vi "VisBx Simulation mit Enum.vi"() -> ()   [LabVIEW 2020, in "Anlagenuebersicht.lvlib"]
uses:
  Anlagenuebersicht.lvlib
  Messwerte.ctl
panel:
  in  "Messwerte":T1
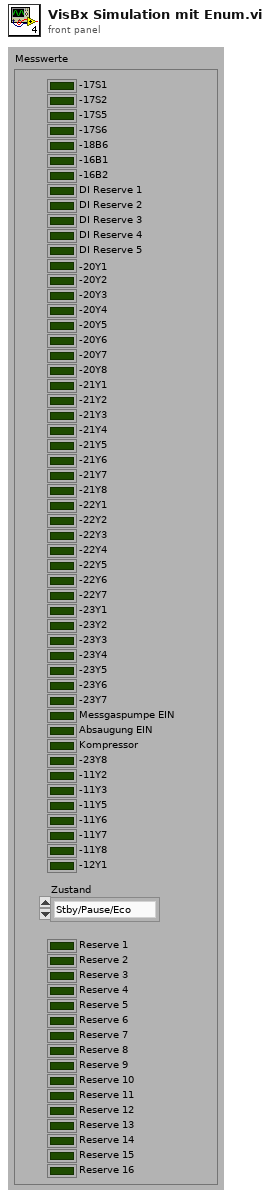
[diagram p1: front panel]
types:
  T1 = typedef "Anlagenuebersicht.lvlib/Messwerte.ctl" = cluster{"-17S1":bool, "-17S2":bool, "-17S5":bool, "-17S6":bool, "-18B6":bool, "-16B1":bool, "-16B2":bool, "DI Reserve 1":bool, "DI Reserve 2":bool, "DI Reserve 3":bool, "DI Reserve 4":bool, "DI Reserve 5":bool, "-20Y1":bool, "-20Y2":bool, "-20Y3":bool, "-20Y4":bool, "-20Y5":bool, "-20Y6":bool, "-20Y7":bool, "-20Y8":bool, "-21Y1":bool, "-21Y2":bool, "-21Y3":bool, "-21Y4":bool, "-21Y5":bool, "-21Y6":bool, "-21Y7":bool, "-21Y8":bool, "-22Y1":bool, "-22Y2":bool, "-22Y3":bool, "-22Y4":bool, "-22Y5":bool, "-22Y6":bool, "-22Y7":bool, "-23Y1":bool, "-23Y2":bool, "-23Y3":bool, "-23Y4":bool, "-23Y5":bool, "-23Y6":bool, "-23Y7":bool, "Messgaspumpe EIN":bool, "Absaugung EIN":bool, "Kompressor":bool, "-23Y8":bool, "-11Y2":bool, "-11Y3":bool, "-11Y5":bool, "-11Y6":bool, "-11Y7":bool, "-11Y8":bool, "-12Y1":bool, "Zustand":enum16{"Stby/Pause/Eco", "Messen", "Spülen Filter", "Spülen Leitung", "Umgebungsluft", "0-Gas / Hintergrund", "Cal-Gas"}, "Reserve 1":bool, "Reserve 2":bool, "Reserve 3":bool, "Reserve 4":bool, "Reserve 5":bool, "Reserve 6":bool, "Reserve 7":bool, "Reserve 8":bool, "Reserve 9":bool, "Reserve 10":bool, "Reserve 11":bool, "Reserve 12":bool, "Reserve 13":bool, "Reserve 14":bool, "Reserve 15":bool, "Reserve 16":bool}
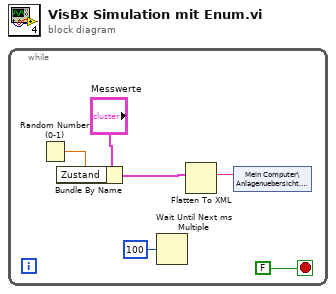
[diagram p0: block diagram]
diagram:
  n1 = while {
    stop <- FALSE stop-if-true
    n2 = Random Number (0-1)() -> (number: 0 to 1=w2:dbl)
    n3 = Bundle By Name(cluster="Messwerte", "Zustand"=w2) -> (w3:T1)
    n4 = Wait Until Next ms Multiple(millisecond multiple=u32 100 ("Vielfache von ms")) -> ()  [unwired: 1 out]
    n5 = Flatten To XML(6:w3) -> (2:w1:string)
    n6 = shared-variable "Mein Computer\\Anlagenuebersicht.lvlib\\VisDat"(w1) -> ()  [unwired: 1 in, 1 out]
  }
